vi "format output buffer.vi"(0 "read buffer":string) -> (12 "Power num":dbl, 13 "Power":string, 14 "In Range?":T2, 15 "Units":string, 16 "Auto Ranging?":T1, 17 "Range W/dBm":T4, 19 "Averaging":T3)   [LabVIEW 2015]
uses:
  Range control watts and dBm.ctl
  Averaging control.ctl
  Range Status.ctl
  Auto Range control.ctl
panel:
  out "Auto Ranging boolean":bool
  out "Averaging?":string
  out "Auto or Hold Range":string
  out "Mode (Unit)":string
  out "Range Status":string
  out "Range Scale":string
  out "substring 2":string
  out "substring":string
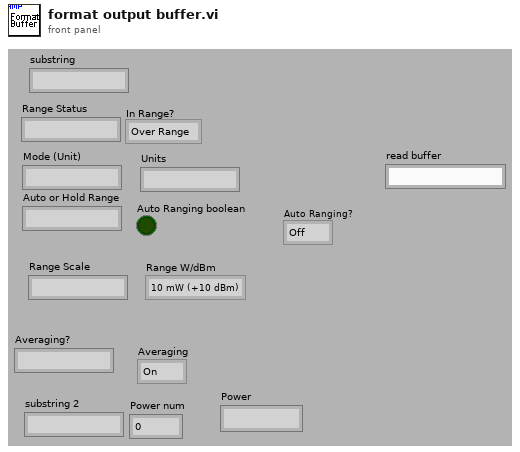
[diagram p1: front panel]
types:
  T1 = typedef "Auto Range control.ctl" = enum16{"Off", "On"}
  T2 = typedef "Range Status.ctl" = enum16{"Over Range", "Under Range", "In Range"}
  T3 = typedef "Averaging control.ctl" = enum16{"On", "Off"}
  T4 = typedef "Range control watts and dBm.ctl" = enum16{"10 mW (+10 dBm)", "1 mW (0 dBm)", "100 uW (-10 dBm)", "10 uW (-20 dBm)", "1 uW (-30 dBm)", "100 nW (-40 dBm)", "10 nW (-50 dBm)", "1 nW (-60 dBm)", "100 pW (-70 dBm)", "10 pW (-80 dBm)"}
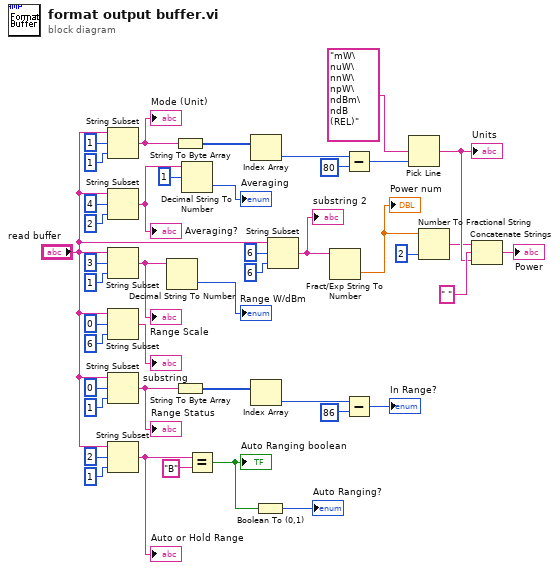
[diagram p0: block diagram]
diagram:
  n1 = String Subset(string="read buffer", offset (0)=1, length (rest)=1 ("length (rest)")) -> (substring=w25:string)
  "Mode (Unit)" <- w25
  n2 = String Subset(string="read buffer", offset (0)=4, length (rest)=2 ("length (rest)")) -> (substring=w18:string)
  "Averaging?" <- w18
  n3 = String Subset(string="read buffer", offset (0)=3, length (rest)=1 ("length (rest)")) -> (substring=w26:string)
  "Range Scale" <- w26
  n4 = String Subset(string="read buffer", offset (0)=0, length (rest)=6 ("length (rest)")) -> (substring=→"substring":string)
  n5 = String Subset(string="read buffer", offset (0)=0, length (rest)=1 ("length (rest)")) -> (substring=w4:string)
  "Range Status" <- w4
  n6 = String Subset(string="read buffer", offset (0)=2, length (rest)=1 ("length (rest)")) -> (substring=w6:string)
  "Auto or Hold Range" <- w6
  n7 = Decimal String To Number(string=w26) -> (number=→"Range W/dBm":i32)  [unwired: 2 in, 1 out]
  n8 = String To Byte Array(string=w25) -> (unsigned byte array=w24:u8[])
  n9 = String To Byte Array(string=w4) -> (unsigned byte array=w15:u8[])
  n10 = Decimal String To Number(string=w18, offset=1) -> (number=→"Averaging":i32)  [unwired: 1 in, 1 out]
  n11 = Equal?(x=w6, y="B") -> (x = y?=w2:bool)
  "Auto Ranging boolean" <- w2
  n12 = Index Array(array=w24) -> (element=w23:u8)  [unwired: 1 in]
  n13 = Index Array(array=w15) -> (element=w14:u8)  [unwired: 1 in]
  n14 = Boolean To (0,1)(Boolean=w2) -> (0, 1=→"Auto Ranging?":i16)
  n15 = String Subset(string="read buffer", offset (0)=6, length (rest)=6 ("length (rest)")) -> (substring=w38:string)
  "substring 2" <- w38
  n16 = Fract/Exp String To Number(string=w38) -> (number=w9:dbl)  [unwired: 3 in, 1 out]
  "Power num" <- w9
  n17 = Subtract(x=w23, y=u8 80) -> (x-y=w20:u8)
  n18 = Subtract(x=w14, y=86) -> (x-y=→"In Range?":i32)
  n19 = Pick Line(multi-line string="mW\nuW\nnW\npW\ndBm\ndB (REL)", line index=w20) -> (output string=w11:string)  [unwired: 1 in]
  "Units" <- w11
  n20 = Number To Fractional String(number=w9, precision (6)=i16 2) -> (F-format string=w8:string)  [unwired: 2 in]
  n21 = Concatenate Strings(w8, " " ("string"), w11) -> (→"Power":string)
